vi "Test.vi"(8 "error in (no error)":errorcluster, 11 "Base Decorator in":refnum<class "Base Decorator.lvclass">) -> (0 "error out":errorcluster, 2 "Pass?":bool, 3 "Base Decorator out":refnum<class "Base Decorator.lvclass">)   [LabVIEW 2020, in "Base Decorator.lvclass"]
uses:
  Base Decorator.lvclass
  Testable/Testable.lvclass
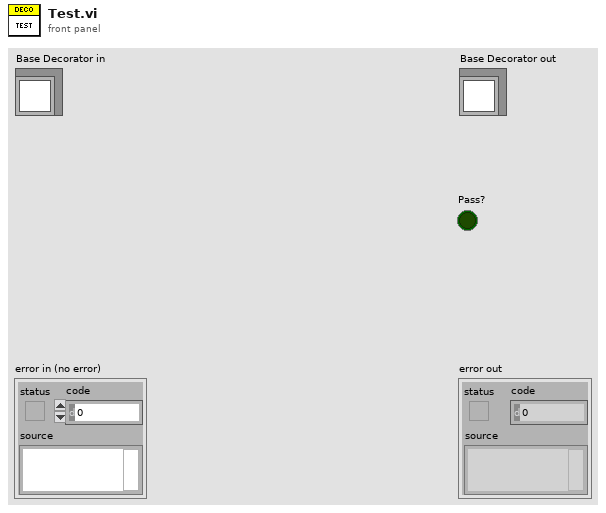
[diagram p1: front panel]
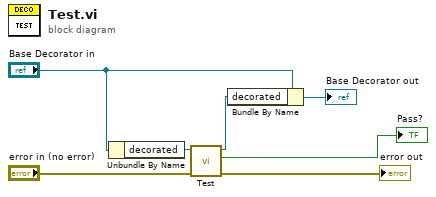
[diagram p0: block diagram]
diagram:
  n1 = Unbundle By Name("Base Decorator in") -> ("decorated"=w7:refnum<class "Testable.lvclass">)
  n2 = call-dynamic "Test.vi"("error in (no error)"="error in (no error)", "Testable in"=w7) -> ("error out"=→"error out":errorcluster, "Pass?"=→"Pass?":bool, "Testable out"=w2:refnum<class "Testable.lvclass">)  [unwired: 7 in]
  n3 = Bundle By Name(cluster="Base Decorator in", "decorated"=w2) -> (→"Base Decorator out":refnum<class "Base Decorator.lvclass">)
